vi "DemoWriteDigital.vi"() -> ()   [LabVIEW 2012]
uses:
  <vilib>/NXT/Block Support/NXT_InputPort.ctl
  <vilib>/NXT/Dual Mode Library/Waits/Wait_Num.vi
  <vilib>/NXT/Dual Mode Library/Waits/Wait_Num(msec).vi
panel:
  in  "stop":bool
  # "Demo Digital Write"
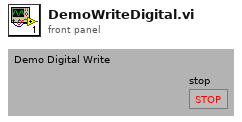
[diagram p1: front panel]
types:
  T1 = typedef "NXT_InputPort.ctl" = u32
  T2 = typedef "LVHSConnector.ctl" = refnum<class "BrickReference.lvclass">
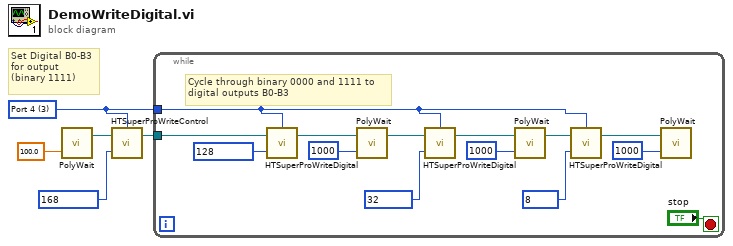
[diagram p0: block diagram]
diagram:
  w4 = T1 3 items=["Port 1", "Port 2", "Port 3", "Port 4"] ("Port")
  # "Set Digital B0-B3\nfor output\n(binary 1111)"
  n1 = call-poly <vilib>:"PolyWait.vi"("Time (1 sec)"=sgl 100.0) -> ("NXT/EV3"=w2:T2)  [unwired: 3 in]
  n2 = call "HTSuperProWriteControl.vi"("Digital Control"=u8 168, "NXT"=w2, "Port"=w4) -> ("NXT"=w5:T2)  [unwired: 2 in]
  n3 = while {
    tunnel: w5 -> [w17]
    tunnel: w4 -> [w6]
    stop <- "stop" stop-if-true
    # "Cycle through binary 0000 and 1111 to\ndigital outputs B0-B3"
    n4 = call "HTSuperProWriteDigital.vi"("Digital Value"=u8 128 ("Digital Control"), "NXT"=w17, "Port"=w6) -> ("NXT"=w16:T2)  [unwired: 2 in]
    n5 = call-poly <vilib>:"PolyWait.vi"("Time (100 msec)"=u32 1000, "NXT/EV3"=w16) -> ("NXT/EV3"=w11:T2)  [unwired: 2 in]
    n6 = call "HTSuperProWriteDigital.vi"("Digital Value"=u8 32 ("Digital Control"), "NXT"=w11, "Port"=w6) -> ("NXT"=w13:T2)  [unwired: 2 in]
    n7 = call-poly <vilib>:"PolyWait.vi"("Time (100 msec)"=u32 1000, "NXT/EV3"=w13) -> ("NXT/EV3"=w7:T2)  [unwired: 2 in]
    n8 = call "HTSuperProWriteDigital.vi"("Digital Value"=u8 8 ("Digital Control"), "NXT"=w7, "Port"=w6) -> ("NXT"=w9:T2)  [unwired: 2 in]
    n9 = call-poly <vilib>:"PolyWait.vi"("Time (100 msec)"=u32 1000, "NXT/EV3"=w9) -> ()  [unwired: 2 in, 1 out]
  }
